vi "core_control_ref_from_name_error_handler.vi"(8 "error in":errorcluster, 9 "control names":string[](array[string]), 10 "found?":bool[](array[boolean]), 11 "vi ref":refnum<vi>) -> (0 "error out":errorcluster, 2 "found? duplicate":bool[](array[boolean]), 3 "vi ref dup":refnum<vi>)   [LabVIEW 2015]
uses:
  polys/poly_ref_tools_eco_plus.vi
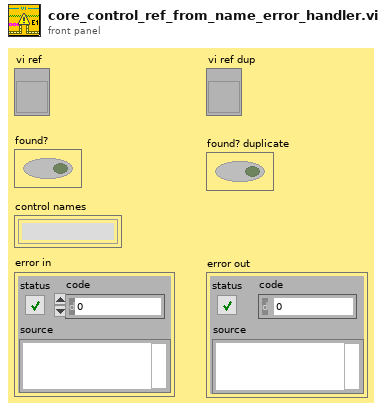
[diagram p1: front panel]
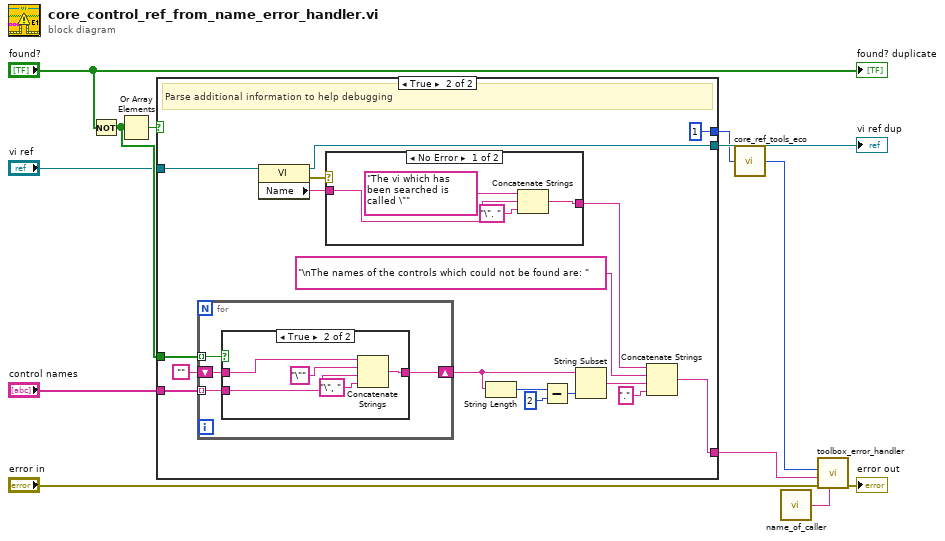
[diagram p0: block diagram]
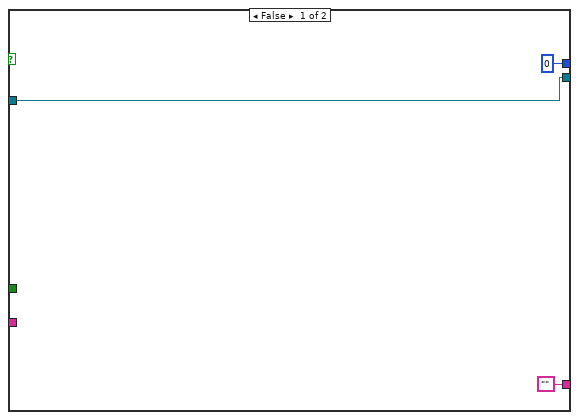
[diagram p2: hidden frame]
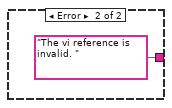
[diagram p3: hidden frame]
diagram:
  n1 = Not(x="found?") -> (.not. x?=w11:bool[])
  n2 = Or Array Elements(Boolean array=w11) -> (logical OR=w12:bool)
  n3 = case shown="True" w12 {
    tunnel: [0 1] -> w6
    tunnel: w11 -> [_ w31]
    tunnel: "control names" -> [_ w30]
    tunnel: ["" w23] -> w2
    tunnel: "vi ref" -> [w13 w22]
    tunnel: [w13 w21] -> w9
    frame False {
    }
    frame True {
      # "Parse additional information to help debugging"
      n4 = for {
        tunnel: w31 -> [w39] mode=indexing
        tunnel: w30 -> [w41] mode=indexing
        shift-right: [w40] -> w27
        shift-left: "" -> [w38]
        n5 = case shown="True" w39 {
          tunnel: w41 -> [_ w47]
          tunnel: [w42 w46] -> w40
          tunnel: w38 -> [w42 w44]
          frame False {
          }
          frame True {
            n6 = Concatenate Strings(w44, "\"", w47, "\", " ("string")) -> (w46:string)
          }
        }
      }
      n7 = property class="VI"(reference=w22) -> (reference out=w21:refnum<vi>, error out=w19:errorcluster, "Name"=w18:string)  [unwired: 1 in]
      n8 = case shown="No Error" w19 {
        tunnel: w18 -> [w35 _]
        tunnel: [w34 "The vi reference is invalid. "] -> w17
        frame No Error {
          n9 = Concatenate Strings("The vi which has been searched is called \"", w35, "\". " ("string")) -> (w34:string)
        }
        frame Error {
        }
      }
      n10 = String Length(string=w27) -> (length=w26:i32)
      n11 = Subtract(x=w26, y=2) -> (x-y=w24:i32)
      n12 = String Subset(string=w27, length (rest)=w24) -> (substring=w28:string)  [unwired: 1 in]
      n13 = Concatenate Strings(w17, "\nThe names of the controls which could not be found are: ", w28, "." ("string")) -> (w23:string)
    }
  }
  "vi ref dup" <- w9
  n14 = call-poly "core_ref_tools_eco.vi"("code (w/out eco)"=w6) -> ("code (+ eco)"=w5:i32)  [unwired: 4 in]
  n15 = call "name_of_caller.vi"() -> ("name of caller out"=w1:string)  [unwired: 4 in]
  n16 = call "toolbox_error_handler.vi"("name of caller in (you)"=w1, "error in (no error)"="error in", "additional info"=w2, "code (0 = no error)"=w5) -> ("error out"=→"error out":errorcluster)  [unwired: 6 in, 1 out]
  "found? duplicate" <- "found?"
